vi "test JSON Error.vi"(8 "error in (no error)":errorcluster, 11 "TestCase in":refnum<class "JSONAble Tests.lvclass">) -> (0 "error out":errorcluster, 3 "TestCase out":refnum<class "JSONAble Tests.lvclass">)   [LabVIEW 2017, in "JSONAble Tests.lvclass"]
uses:
  JSONAble Tests.lvclass
  Classes/error/error.lvclass
  Classes/error/error.Write code.vi
  Classes/error/error.Write data.vi
  Classes/error/error.Write message.vi
  <vilib>/addons/_JKI Toolkits/VI Tester/TestCase.llb/TestCase.lvclass
  <vilib>/National Instruments/Variant JSON API/Variant JSON API.lvlib
  C:/Program Files (x86)/National Instruments/LabVIEW 2017/vi.lib/addons/_JKI Toolkits/VI Tester/TestCase.llb/TestCase.lvclass
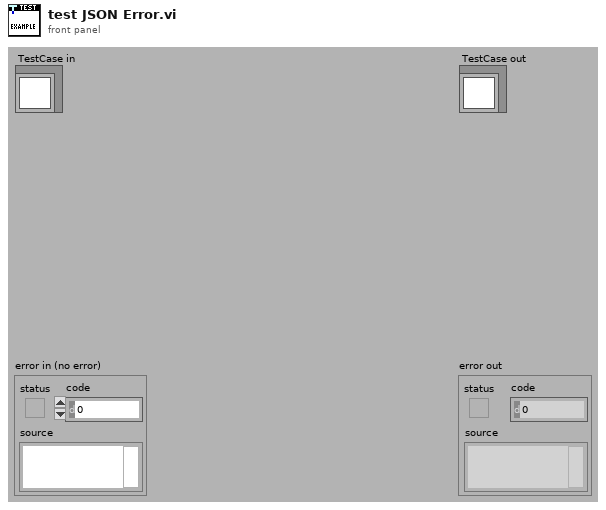
[diagram p1: front panel]
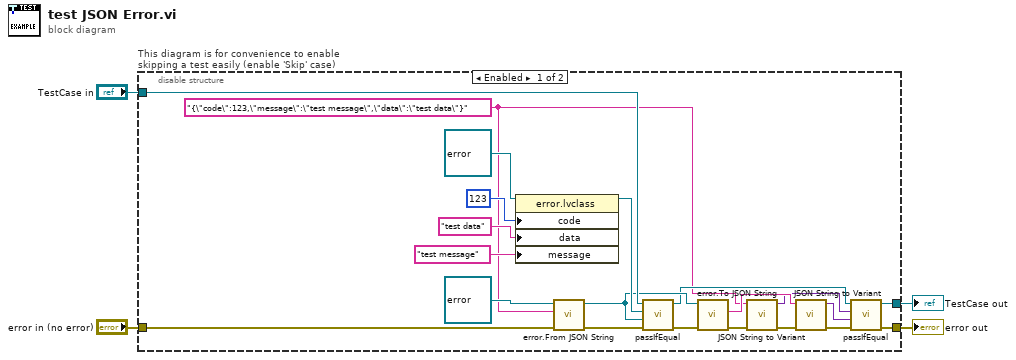
[diagram p0: block diagram]
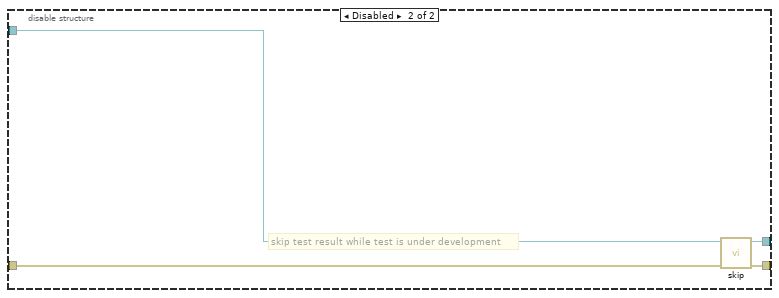
[diagram p2: hidden frame]
diagram:
  n1 = disable-structure "This diagram is for convenience to enable skipping a test easily (enable 'Skip' case)" shown="Enabled" {
    disable-tunnel: "TestCase in" -> [w20 w29]
    disable-tunnel: [w12 w27] -> w1
    disable-tunnel: [w14 w28] -> w3
    disable-tunnel: "error in (no error)" -> [w18 w26]
    frame Enabled {
      w10 = "{\"code\":123,\"message\":\"test message\",\"data\":\"test data\"}" ("JSON String")
      n2 = property class="error.lvclass"(reference=refnum<class "error.lvclass"> refnum ("error.lvclass"), "code"=123, "data"="test data" ("message"), "message"="test message") -> (reference out=w19:refnum<class "error.lvclass">)  [unwired: 1 in, 1 out]
      n3 = call "error.From JSON String.vi"("error in (no error)"=w18, "JSON String"=w10, "error in"=refnum<class "error.lvclass"> refnum ("error.lvclass")) -> (0:"error out"=w16:errorcluster, 3:"error out"=w17:refnum<class "error.lvclass">)  [unwired: 7 in]
      n4 = call-dynamic "passIfEqual.vi"("error in (no error)"=w16, "y"=w17, "x"=w19, "TestCase in"=w20) -> ("error out"=w15:errorcluster, "TestCase out"=w13:refnum<class "JSONAble Tests.lvclass">)  [unwired: 6 in]
      n5 = call "error.To JSON String.vi"("error in (no error)"=w15, "error in"=w17) -> ("error out"=w7:errorcluster, "JSON String"=w11:string)  [unwired: 7 in, 1 out]
      n6 = call <vilib>:"JSON String to Variant.vi"("error in (no error)"=w7, "JSON String"=w10) -> ("error out"=w6:errorcluster, "Variant out"=w8:variant)  [unwired: 8 in]
      n7 = call <vilib>:"JSON String to Variant.vi"("error in (no error)"=w6, "JSON String"=w11) -> ("error out"=w5:errorcluster, "Variant out"=w9:variant)  [unwired: 8 in]
      n8 = call-dynamic "passIfEqual.vi"("error in (no error)"=w5, "y"=w9, "x"=w8, "TestCase in"=w13) -> ("error out"=w14:errorcluster, "TestCase out"=w12:refnum<class "JSONAble Tests.lvclass">)  [unwired: 6 in]
    }
    frame Disabled {
      # "skip test result while test is under development"
      n9 = call <vilib>:"skip.vi"("error in (no error)"=w26, "TestCase in"=w29) -> ("error out"=w28:errorcluster, "TestCase out"=w27:refnum<class "JSONAble Tests.lvclass">)  [unwired: 8 in]
    }
  }
  "error out" <- w3
  "TestCase out" <- w1
